vi "Initialize From Settings.vi"(8 "error in (no error)":errorcluster, 10 "settings":cluster{"key":string, "value":string}[](array[cluster]), 11 "User Interface in":refnum<class "User Interface.lvclass">) -> (0 "error out":errorcluster, 3 "User Interface out":refnum<class "User Interface.lvclass">)   [LabVIEW 2020, in "DSF Core.lvlib" / "User Interface.lvclass"]
uses:
  User Interface.lvclass
  User Interface.lvclass/User Interface.ctl
  Configuration/Configuration.lvclass
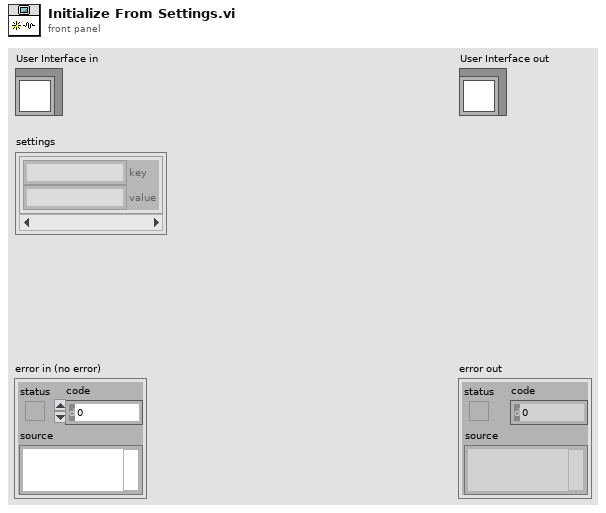
[diagram p1: front panel]
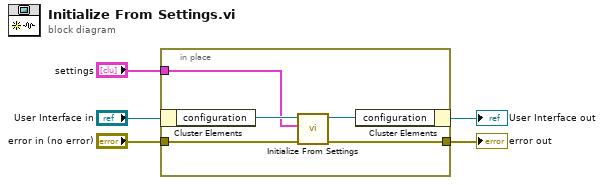
[diagram p0: block diagram]
diagram:
  n1 = in-place {
    in-place-border: "error in (no error)" -> [w8]
    in-place-border: [w7] -> w2
    in-place-border: "settings" -> [w6]
    n2 = in-place-cluster #1("User Interface in") -> ("configuration"=w10:refnum<class "Configuration.lvclass">)
    n3 = call-dynamic "Initialize From Settings.vi"("error in (no error)"=w8, "settings"=w6, "Configuration in"=w10) -> ("error out"=w7:errorcluster, "Configuration out"=w9:refnum<class "Configuration.lvclass">)  [unwired: 7 in]
    n4 = in-place-cluster #1("configuration"=w9) -> (→"User Interface out":refnum<class "User Interface.lvclass">)
  }
  "error out" <- w2
